vi "Image Queue.vi"(6 "timeout in ms (-1)":i32, 7 "Action":T2=enum."Enqueue", 8 "Error In":errorcluster, 11 "Image In":T1) -> (0 "Error Out":errorcluster, 3 "Image Out":T1)   [LabVIEW 2018]
uses:
  Controls/Queue Manager Actions.ctl
  <vilib>/vision/Image Controls.llb/IMAQ Image.ctl
  Controls/MessagePacket.ctl
  Controls/QueueNames.ctl
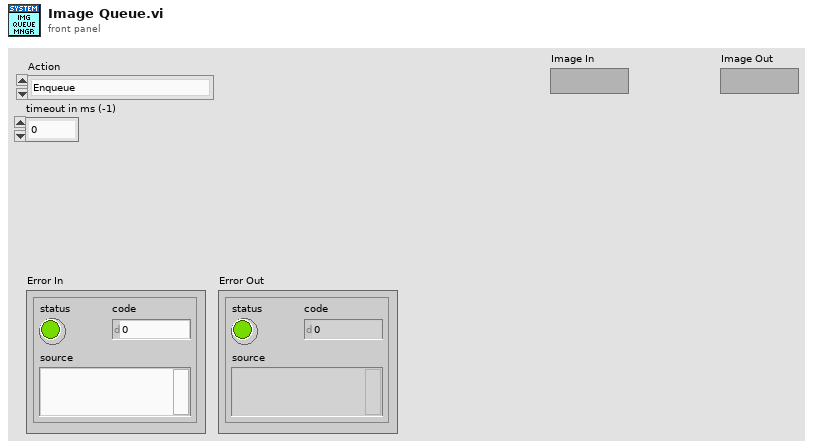
[diagram p1: front panel]
types:
  T1 = typedef "IMAQ Image.ctl" = refnum<image>
  T2 = typedef "Queue Manager Actions.ctl" = enum16{"Init", "Enqueue", "Enqueue All", "Preview Queue", "Dequeue", "Get Status", "Flush Queue", "Flush All Queues", "Release All Queues", "Release Queue", "Enqueue at Opposite End"}
  T3 = typedef "MessagePacket.ctl" = cluster{"Message":string, "Parameter":variant}
  T4 = typedef "QueueNames.ctl" = enum16{"Main GUI", "Main Scan Processor", "Main Processing", "Main Saving", "Main Display", "Main Table Stage GUI", "Main Table Stage Proc.", "Scan Engine", "Vibratome GUI", "Vibratome Processor", "Slice Engine"}
  T5 = typedef "Image Type" = u32
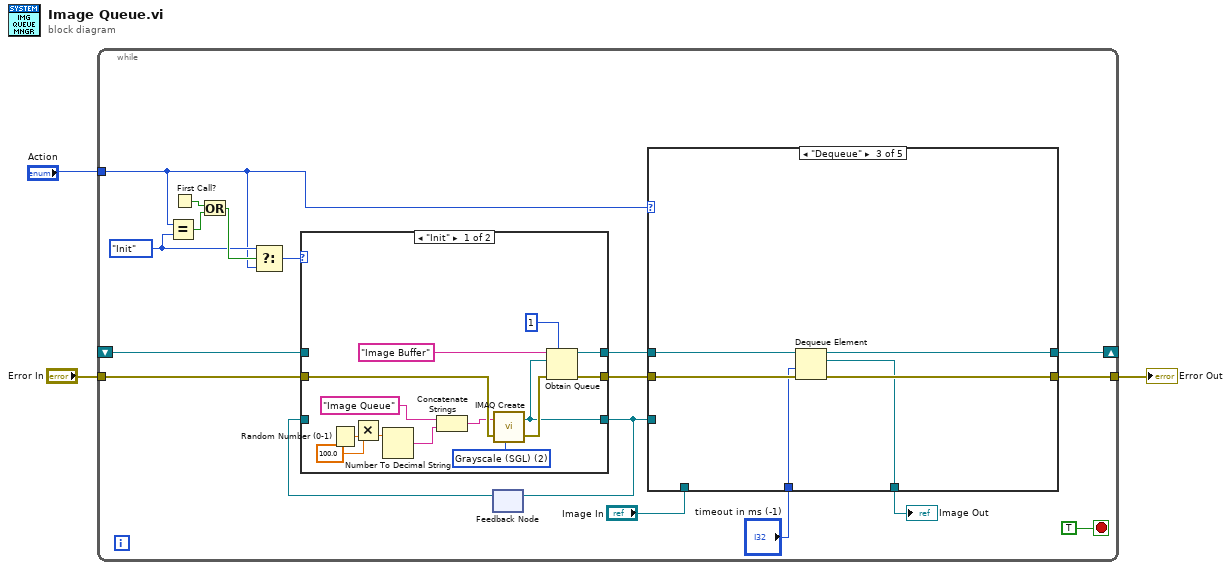
[diagram p0: block diagram]
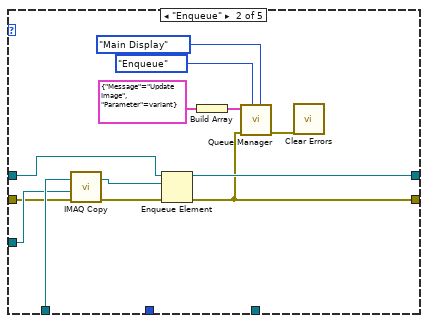
[diagram p3: hidden frame]
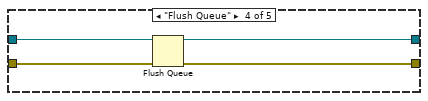
[diagram p4: hidden frame]
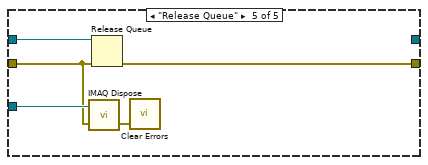
[diagram p5: hidden frame]
diagram:
  n1 = while {
    tunnel: "Action" -> [w9]
    tunnel: "Error In" -> [w16]
    tunnel: [w15] -> w1
    shift-right: [w11] -> _
    shift-left: _ -> [w10]
    stop <- TRUE stop-if-true
    w18 = Queue_Manager_Actions."Init"
    n2 = Equal?(x=w9, y=w18) -> (x = y?=w20:bool)
    n3 = First Call?() -> (First Call?: T/F=w21:bool)
    n4 = Or(x=w21, y=w20) -> (x .or. y?=w19:bool)
    n5 = Select(t=w18, s=w19, f=w9) -> (s? t:f=w17:T2)
    n6 = feedback #1() -> (w6:T1)  [unwired: 1 in]
    n7 = case shown="\"Init\"" w17 {
      tunnel: [w65 w67] -> w13
      tunnel: w16 -> [w60 w68]
      tunnel: [w64 w68] -> w14
      tunnel: w10 -> [_ w67]
      tunnel: [w59 w66] -> w7
      tunnel: w6 -> [_ w66]
      frame "Init" {
        w53 = T5 2 items=["Grayscale (U8)", "Grayscale (I16)", "Grayscale (SGL)", "Complex (CSG)", "RGB (U32)", "HSL (U32)", "RGB (U64)", "Grayscale (U16)"] ("Image Type")
        n8 = Random Number (0-1)() -> (number: 0 to 1=w55:dbl)
        n9 = Multiply(x=100.0, y=w55) -> (x*y=w56:dbl)
        n10 = Number To Decimal String(number=w56) -> (decimal integer string=w54:string)  [unwired: 1 in]
        n11 = Concatenate Strings("Image Queue" ("Image Name"), w54) -> (w58:string)
        n12 = call "IMAQ Create"("Image Name"=w58, "Image Type"=w53, "error in (no error)"=w60) -> ("New Image"=w59:T1, "error out"=w61:errorcluster)  [unwired: 2 in]
        n13 = Obtain Queue(max queue size (-1, unlimited)=1, name (unnamed)="Image Buffer", element data type=w59, error in (no error)=w61) -> (queue out=w65:refnum<queue>, error out=w64:errorcluster)  [unwired: 1 in, 1 out]
      }
      frame "Enqueue", Default {
      }
    }
    n14 = feedback-in #1(w7) -> ()
    n15 = case shown="\"Dequeue\"" w9 {
      tunnel: w13 -> [w22 w32 w39 w44 w50]
      tunnel: [w23 w25 w41 w45 w51] -> w15
      tunnel: w14 -> [w23 w34 w42 w46 w48]
      tunnel: [_ _ w40 _ _] -> w8
      tunnel: [w22 w30 w38 w43 _] -> w11
      tunnel: w7 -> [_ w35 _ _ w49]
      tunnel: "Image In" -> [_ w36 _ _ _]
      tunnel: "timeout in ms (-1)" -> [_ _ w37 _ _]
      frame "Init", Default {
      }
      frame "Enqueue" {
        n16 = call "IMAQ Copy"("error in (no error)"=w34, "Image Dst"=w35, "Image Src"=w36) -> ("error out"=w33:errorcluster, "Image Dst Out"=w31:T1)  [unwired: 3 in]
        n17 = Enqueue Element(queue=w32, element=w31, error in (no error)=w33) -> (queue out=w30:refnum<queue>, error out=w25:errorcluster)  [unwired: 1 in, 1 out]
        n18 = Build Array(T3 {"Message"="Update Image", "Parameter"=variant} ("Message Packet [In]")) -> (w26:T3[])
        n19 = call "Queue Manager.vi"("Queue Name"=QueueNames."Main Display", "Action"=Queue_Manager_Actions."Enqueue", "Error In"=w25, "Message Packet Array"=w26) -> ("Error Out"=w24:errorcluster)  [unwired: 3 in, 4 out]
        n20 = call <vilib>:"Clear Errors.vi"("error in (no error)"=w24) -> ()  [unwired: 5 in, 2 out]
      }
      frame "Dequeue" {
        n21 = Dequeue Element(queue=w39, timeout in ms (-1)=w37, error in (no error)=w42) -> (queue out=w38:refnum<queue>, element=w40:T1, error out=w41:errorcluster)  [unwired: 1 out]
      }
      frame "Flush Queue" {
        n22 = Flush Queue(queue=w44, error in (no error)=w46) -> (queue out=w43:refnum<queue>, error out=w45:errorcluster)  [unwired: 1 out]
      }
      frame "Release Queue" {
        n23 = call "IMAQ Dispose"("Image"=w49, "error in (no error)"=w48) -> ("error out"=w47:errorcluster)  [unwired: 4 in]
        n24 = Release Queue(queue=w50, error in (no error)=w48) -> (error out=w51:errorcluster)  [unwired: 1 in, 2 out]
        n25 = call <vilib>:"Clear Errors.vi"("error in (no error)"=w47) -> ()  [unwired: 5 in, 2 out]
      }
    }
    "Image Out" <- w8
  }
  "Error Out" <- w1
